vi "Camera_Config.vi"(5 "Crop?":bool, 6 "Camera":T5, 7 "error in":errorcluster, 8 "input cluster":T1={"Pinch-valve"="Test Sample", "XLP 6000 Pump"="MRJ", "Camera1"="", "Camera2"="", "Img_Capt"=FALSE, "Actuator"=FALSE, "Pump"=FALSE, "Cam 1"=FALSE, "Cam 2"=FALSE, "Empty_Refill"=FALSE, "Crop"=FALSE, "Light intensity"=0, "Exposure Time"=0.0, "Sample Name"="", "Operator"="", "Calibration 1"=path "C:/Users/au540322/Desktop/IHS_Project/images/Debris/Debris_0/Debris_0_2019_06_01-23-32-49-686.PNG", "Calibration 2"=path "C:/Users/au540322/Desktop/IHS_Project/images/Debris/Debris_0/Debris_0_2019_06_01-23-32-49-686.PNG", "Framerate"=1, "Timeout Sample"=1, "Collection date"="", "Sample size threshold"=500, "Empty start"=500, "Command"="", "Station"="", "Species Name"="", "Other Notes"="", "Aperture"=enum."Item 3", "Image Process Queue Size"=100, "Image Save Queue Size"=0, "Overload threshold"=0, "Max Framerate"=0, "Rectangle 1"={"Left"=0, "Top"=0, "Right"=0, "Bottom"=0, "Rotation"=0.0}, "Rectangle 2"={"Left"=0, "Top"=100, "Right"=100, "Bottom"=0, "Rotation"=0.0}, "Detection Region %"=200.0, "Detect 1"=path "C:/Users/au540322/Desktop/IHS_Project/images/Debris/Debris_0/Debris_0_2019_06_01-23-32-49-686.PNG", "Detect 2"=path "C:/Users/au540322/Desktop/IHS_Project/images/Debris/Debris_0/Debris_0_2019_06_01-23-32-49-686.PNG", "Max large object threshold"=500, "Open(T)/Close(F)"=FALSE, "Img_Capt Begin"=FALSE, "Dispense Speed"=0, "Flush Size"=0, "Location"="", "Latitude"="", "Longitude"="", "Determiner"="", "Sex"="", "Camera1_Img"=refnum, "Camera2_Img"=refnum, "Img1_Orig_Disp"=refnum, "Img2_Orig_Disp"=refnum, "Img1_Orig_RGB"=refnum, "Img2_Orig_RGB"=refnum, "Blue_Plane_Extract"=refnum, "Subtracted_Plane"=refnum, "Img1_Binary"=refnum, "Img2_Binary"=refnum, "Crop_Mask"=refnum, "Img1_Save"=refnum, "Img2_Save"=refnum, "Img1_Cali_Full"=refnum, "Img2_Cali_Full"=refnum, "Img1_Cali_Detect"=refnum, "Img2_Cali_Detect"=refnum, "Cam 1 queue"=refnum, "Cam 2 queue"=refnum, "Cam 1 - save queue"=refnum, "Cam 2 - save queue"=refnum, "Overlay_Ring"=0, "SystemVersion"=0, "System Serial"="", "Legacy Cam Attributes"=FALSE, "Camera Orientation 1"="", "Camera Orientation 2"="", "Pixel to mm 1"=0.0, "Pixel to mm 2"=0.0, "CAM1 Model"=enum."a2A5328-15ucBAS", "CAM2 Model"=enum."a2A5328-15ucBAS", "Flush Insect"=FALSE, "Pump Size"=FALSE, "Barcode"="", "Phase3"=FALSE, "Mega F3"="", "Container nr."=0.0, "Mannual F3"=TRUE} {"SystemVersion" items=["Standard", "XL"]; "Overlay_Ring" items=["Session Data", "Extended Setup", "Buffer", "Camera", "Dispenser", "Stats", "Connections"]; "Flush Size" min=1; "Dispense Speed" min=1; "Rectangle 2"."Rotation" format="%.2f"; "Rectangle 2"."Left" scale=0.0..1024.0; "Rectangle 2"."Right" scale=0.0..1024.0; "Rectangle 1"."Rotation" format="%.2f"; "Rectangle 1"."Left" scale=0.0..1024.0; "Rectangle 1"."Right" scale=0.0..1024.0; "Max Framerate" min=1; "Overload threshold" min=1; "Image Save Queue Size" min=1; "Image Process Queue Size" min=1; "Empty start" min=1; "Sample size threshold" min=1; "Framerate" min=1; "Light intensity" scale=0.0..100.0}, 9 "Detect Movement":bool, 10 "Refnum in":T2="cam2") -> (0 "error out":errorcluster, 3 "Refnum out":T2="cam2")   [LabVIEW 2024]
doc: "Configures basler cameras for image acquisition with cropped aspectratio."
uses:
  <vilib>/userDefined/High Color/IMAQdx.ctl
  Camera_ID.ctl
  controls/Data.ctl
  <vilib>/vision/Image Controls.llb/IMAQ Image.ctl
panel:
  out "error out 2":errorcluster
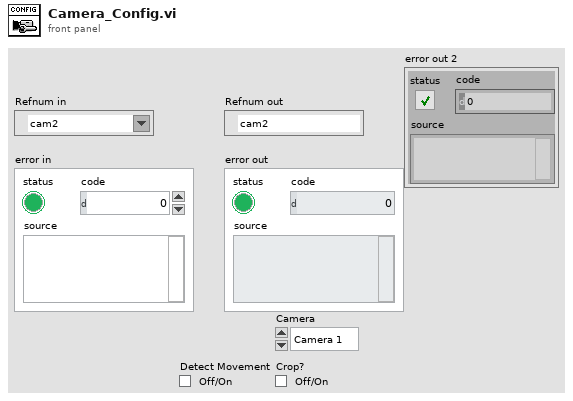
[diagram p1: front panel]
types:
  T1 = typedef "Data.ctl" = cluster{"Pinch-valve":refnum<visa-resource-name>, "XLP 6000 Pump":refnum<visa-resource-name>, "Camera1":T2, "Camera2":T2, "Img_Capt":bool, "Actuator":bool, "Pump":bool, "Cam 1":bool, "Cam 2":bool, "Empty_Refill":bool, "Crop":bool, "Light intensity":i32, "Exposure Time":dbl, "Sample Name":string, "Operator":string, "Calibration 1":path, "Calibration 2":path, "Framerate":i32, "Timeout Sample":i32, "Collection date":string, "Sample size threshold":i32, "Empty start":u32, "Command":string, "Station":string, "Species Name":string, "Other Notes":string, "Aperture":enum32{"Item 0", "Item 1", "Item 2", "Item 3"}, "Image Process Queue Size":i32, "Image Save Queue Size":i32, "Overload threshold":i32, "Max Framerate":i32, "Rectangle 1":T3, "Rectangle 2":T3, "Detection Region %":dbl, "Detect 1":path, "Detect 2":path, "Max large object threshold":i32, "Open(T)/Close(F)":bool, "Img_Capt Begin":bool, "Dispense Speed":i32, "Flush Size":i32, "Location":string, "Latitude":string, "Longitude":string, "Determiner":string, "Sex":string, "Camera1_Img":T4, "Camera2_Img":T4, "Img1_Orig_Disp":T4, "Img2_Orig_Disp":T4, "Img1_Orig_RGB":T4, "Img2_Orig_RGB":T4, "Blue_Plane_Extract":T4, "Subtracted_Plane":T4, "Img1_Binary":T4, "Img2_Binary":T4, "Crop_Mask":T4, "Img1_Save":T4, "Img2_Save":T4, "Img1_Cali_Full":T4, "Img2_Cali_Full":T4, "Img1_Cali_Detect":T4, "Img2_Cali_Detect":T4, "Cam 1 queue":refnum<queue>, "Cam 2 queue":refnum<queue>, "Cam 1 - save queue":refnum<queue>, "Cam 2 - save queue":refnum<queue>, "Overlay_Ring":u16, "SystemVersion":u16, "System Serial":string, "Legacy Cam Attributes":bool, "Camera Orientation 1":string, "Camera Orientation 2":string, "Pixel to mm 1":dbl, "Pixel to mm 2":dbl, "CAM1 Model":enum16{"a2A5328-15ucBAS", "acA1920-155uc"}, "CAM2 Model":enum16{"a2A5328-15ucBAS", "acA1920-155uc"}, "Flush Insect":bool, "Pump Size":bool, "Barcode":string, "Phase3":bool, "Mega F3":refnum<visa-resource-name>, "Container nr.":dbl, "Mannual F3":bool}
  T2 = typedef "IMAQdx.ctl" = refnum<k21>
  T3 = typedef "IMAQ Rectangle" = cluster{"Left":i32, "Top":i32, "Right":i32, "Bottom":i32, "Rotation":dbl}
  T4 = typedef "IMAQ Image.ctl" = refnum<image>
  T5 = typedef "Camera_ID.ctl" = enum16{"Camera 1", "Camera 2"}
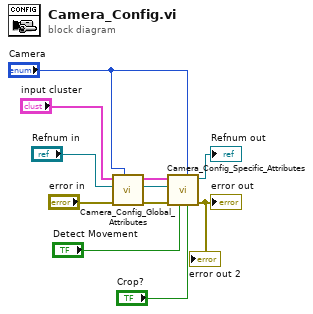
[diagram p0: block diagram]
diagram:
  n1 = call "Camera_Config_Global_Attributes.vi"("Camera"="Camera", "error in (no error)"="error in", "Refnum in"="Refnum in", "input cluster"="input cluster") -> ("error out"=w8:errorcluster, "Refnum out"=w4:T2, "input cluster out"=w3:T1)  [unwired: 5 in]
  n2 = call "Camera_Config_Specific_Attributes.vi"("Crop?"="Crop?", "Camera"="Camera", "Detect Movement"="Detect Movement", "error in (no error)"=w8, "Refnum in"=w4, "input cluster"=w3) -> ("error out"=→"error out" →"error out 2":errorcluster, "Refnum out"=→"Refnum out":T2)  [unwired: 4 in]
